vi "Write Class Instance.vi"(8 "error in (no error)":errorcluster, 10 "Instance":refnum<class>, 11 "Test Runner.Project in":refnum<class "Test Runner.Class.lvclass">) -> (0 "error out":errorcluster, 3 "Test Runner.Project out":refnum<class "Test Runner.Class.lvclass">)   [LabVIEW 2020, in "Caraya.lvlib" / "Test Runner.Class.lvclass"]
uses:
  Test Runner.Class.lvclass
  Test Runner.Class.lvclass/Test Runner.Class.ctl
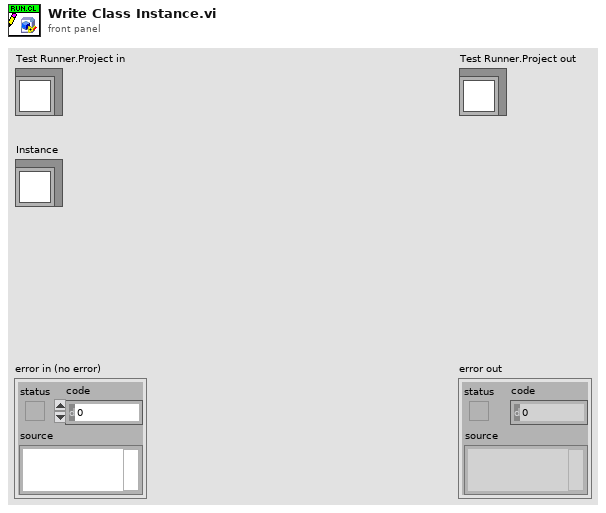
[diagram p1: front panel]
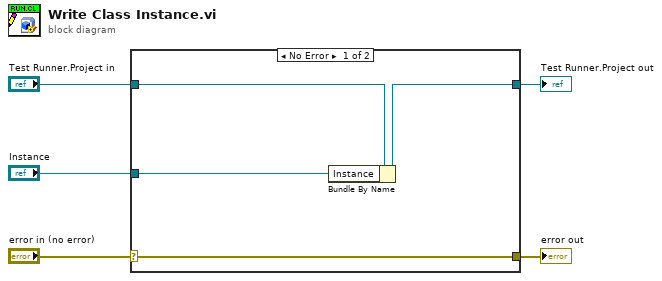
[diagram p0: block diagram]
diagram:
  n1 = case shown="No Error" "error in (no error)" {
    selector: "error in (no error)" -> [w9 w10]
    tunnel: [w9 w10] -> w4
    tunnel: [w6 w11] -> w2
    tunnel: "Test Runner.Project in" -> [w8 w11]
    tunnel: "Instance" -> [w7 _]
    frame No Error {
      n2 = Bundle By Name(cluster=w8, "Instance"=w7) -> (w6:refnum<class "Test Runner.Class.lvclass">)
    }
    frame Error {
    }
  }
  "error out" <- w4
  "Test Runner.Project out" <- w2
